vi "Create PID.vi"(7 "Input?":bool, 8 "error in (no error)":errorcluster, 10 "DIDPID":T2 {"Signals"."Byte Order" items=["Little Endian", "Big Endian"]; "Signals"."Data Type" items=["Signed", "Unsigned", "IEEE Float"]}, 11 "Section Ptr":T1 format="%.0x") -> (0 "error out":errorcluster, 3 "Parent Ref out":T1 format="%.0x")   [LabVIEW 2015, in "Diagnostics Addon Shared.lvlib"]
uses:
  Diagnostics Addon Shared.lvlib
  DIDPID Parameters.ctl
  DIDPID Signal Parameters.ctl
  <vilib>/NI Veristand/Custom Device API/Custom Device Item Ref.ctl
  GUID Lookup.vi
  <vilib>/NI Veristand/Custom Device API/Custom Device API.lvlib
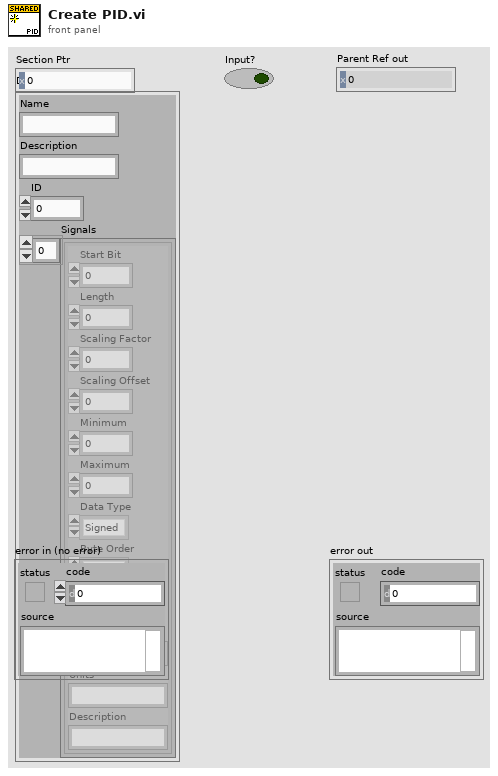
[diagram p1: front panel]
types:
  T1 = typedef "Custom Device API.lvlib/Custom Device Item Ref.ctl" = u64
  T2 = typedef "Diagnostics Addon Shared.lvlib/DIDPID Parameters.ctl" = cluster{"Name":string, "Description":string, "ID":u16, "Signals":T3[]}
  T3 = typedef "Diagnostics Addon Shared.lvlib/DIDPID Signal Parameters.ctl" = cluster{"Start Bit":u8, "Length":u8, "Scaling Factor":dbl, "Scaling Offset":dbl, "Minimum":dbl, "Maximum":dbl, "Data Type":u32, "Byte Order":u32, "Default Value":dbl, "Name":string, "Units":string, "Description":string}
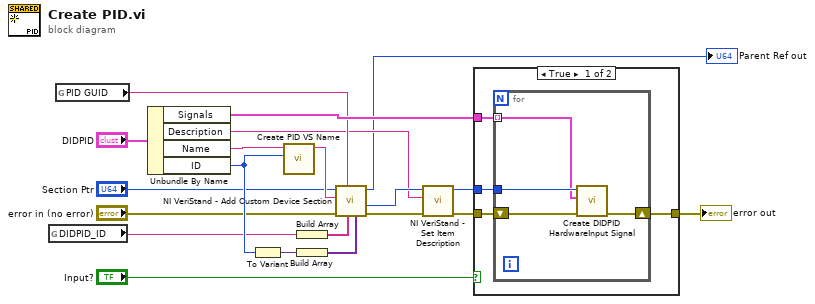
[diagram p0: block diagram]
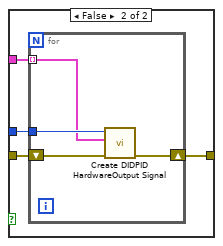
[diagram p2: hidden frame]
diagram:
  n1 = global read "GUID Lookup.vi" "DIDPID_ID"() -> (w13:string)
  n2 = global read "GUID Lookup.vi" "PID GUID"() -> (w10:string)
  n3 = Unbundle By Name("DIDPID") -> ("Signals"=w17:T3[], "Description"=w2:string, "Name"=w18:string, "ID"=w19:u16)
  n4 = To Variant(anything=w19) -> (Variant=w14:variant)
  n5 = call "Create PID VS Name.vi"("PID Number"=w19, "PID Name"=w18) -> ("VS Name"=w20:string)  [unwired: 9 in]
  n6 = Build Array(w13) -> (w12:string[])
  n7 = Build Array(w14) -> (w15:variant[])
  n8 = call <vilib>:"NI VeriStand - Add Custom Device Section.vi"("Property Values"=w15, "Property names"=w12, "GUID (Default Section)"=w10, "error in (no error)"="error in (no error)", "Section Name"=w20, "Parent Ref in"="Section Ptr") -> ("error out"=w8:errorcluster, "Section Ptr"=w6:T1, "Parent Ref out"=→"Parent Ref out":T1)  [unwired: 2 in, 1 out]
  n9 = call <vilib>:"NI VeriStand - Set Item Description.vi"("error in (no error)"=w8, "Description"=w2, "Item Ref in"=w6) -> ("error out"=w7:errorcluster, "Item Ref out"=w5:T1)  [unwired: 6 in, 1 out]
  n10 = case shown="True" "Input?" {
    tunnel: w5 -> [w24 w32]
    tunnel: w17 -> [w23 w31]
    tunnel: [w22 w30] -> w16
    tunnel: w7 -> [w21 w29]
    frame True {
      n11 = for {
        shift-right: [w27] -> w22
        shift-left: w21 -> [w28]
        tunnel: w23 -> [w25] mode=indexing
        tunnel: w24 -> [w26]
        n12 = call "Create DIDPID HardwareInput Signal.vi"("error in (no error)"=w28, "Signal Parameters"=w25, "Section Ptr"=w26) -> ("error out"=w27:errorcluster)  [unwired: 7 in, 1 out]
      }
    }
    frame False {
      n13 = for {
        shift-right: [w33] -> w30
        shift-left: w29 -> [w35]
        tunnel: w31 -> [w34] mode=indexing
        tunnel: w32 -> [w36]
        n14 = call "Create DIDPID HardwareOutput Signal.vi"("error in (no error)"=w35, "Signal Parameters"=w34, "Section Ptr"=w36) -> ("error out"=w33:errorcluster)  [unwired: 7 in, 1 out]
      }
    }
  }
  "error out" <- w16
